vi "Array - Failure Message.vi"() -> ()   [LabVIEW 2017, in "Transparent Assertions.Tests.lvlib" / "Assert Collection Not Empty.lvlib"]
uses:
  Assert Collection Not Empty.lvlib
  src/Transparent Assertions/Transparent Assertions.lvlib
panel:
  out "error out":errorcluster
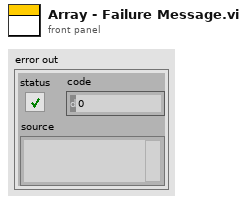
[diagram p1: front panel]
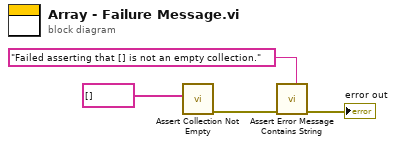
[diagram p0: block diagram]
diagram:
  n1 = call "Assert Collection Not Empty.vi"("Collection"=string[] []) -> ("error out"=w2:errorcluster)  [unwired: 10 in]
  n2 = call "Assert Error Message Contains String.vi"("Expected"="Failed asserting that [] is not an empty collection.", "error in (no error)"=w2) -> ("error out"=→"error out":errorcluster)  [unwired: 9 in]
